vi "svc_FFT with Window.vi"(0 "time signal in [EU]":waveform(dbl), 2 "window":T1=1 items=["None"=0, "Hanning"=1, "Hamming"=2, "Blackman-Harris"=3, "Exact Blackman"=4, "Blackman"=5, "Flat Top"=6, "4 Term B-Harris "=7, "7 Term B-Harris"=8, "Low Sidelobe"=9, "Force"=64, "Exponential"=65, "Blackman Nuttall"=11, "Triangle"=30, "Bartlett-Hanning"=31, "Bohman"=32, "Parzen"=33, "Welch"=34, "Kaiser"=60, "Dolph-Chebyshev"=61, "Gaussian"=62], 5 "error in (no error)":errorcluster) -> (14 "complex spectrum":T8={"complex spectrum response"={"f0"=0.0, "df"=1.0, "complex spectrum"=[]}, "spectrum info"={"channel name"="", "description"="", "x-axis units"=0, "spectral info"={"spectrum type"=enum."Power [Magnitude^2]", "linear/dB"=enum."linear", "window"=0, "window size"=0, "FFT size"=0}, "engineering units"=0, "custom label"="", "dB reference [EU]"=0.0, "peak units"=enum."rms", "weighting filter"=0, "spectral density?"=FALSE, "unit label"="", "spectrum skewed?"=FALSE, "complimentary spectrum units"=enum."none"}} {"spectrum info"."x-axis units" items=["Time (s)"=0, "Frequency-CB (Hz)"=1, "Frequency-CPB (Hz)"=1248, "Frequency-Arbitrary (Hz)"=2357, "Quefrency (s)"=2, "Revolutions (rev)"=3, "Order"=4, "Speed (RPM)"=11, "Speed (rad/s)"=21, "Index"=65535]; "spectrum info"."weighting filter" items=["Linear", "A-weighting", "B-weighting", "C-weighting", "ITU-R 468-4", "Dolby", "CCITT", "C-message", "Wb", "Wc", "Wd", "We", "Wf", "Wh", "Wj", "Wk", "Wm", "AES17 20 kHz lowpass", "AES17 40 kHz lowpass", "AES17 20 kHz highpass", "AES17 40 kHz highpass"]; "spectrum info"."dB reference [EU]" format="%.2f"; "spectrum info"."engineering units" items=["custom..."=0, "V"=1, "A"=21, "C"=30, "pC"=31, "s"=32, "-"=29, "Pa"=2, "N"=20, "g"=3, "m/s^2"=4, "m/s"=5, "m"=6, "mm/s"=12, "mm"=13, "micron/s"=14, "micron"=15, "in/s^2"=7, "in/s"=8, "in"=9, "mil/s"=10, "mil"=11, "rad/s^2"=16, "rad/s"=17, "rad"=18, "deg/s^2"=26, "deg/s"=27, "deg"=28, "RPM"=22, "cycle/s^2"=23, "Hz"=24, "cycle"=25, "strain"=19]; "spectrum info"."spectral info"."window" items=["None "=0, "Hanning"=1, "Hamming"=2, "Blackman-Harris"=3, "Exact Blackman"=4, "Blackman"=5, "Flat Top"=6, "4 Term B-Harris "=7, "7 Term B-Harris"=8, "Low Sidelobe"=9, "Force - Exponential"=10, "Gaussian"=62]; "complex spectrum response"."complex spectrum" format="%.2f"; "complex spectrum response"."df" format="%.2f"; "complex spectrum response"."f0" format="%.2f"}, 19 "error out":errorcluster)   [LabVIEW 2017]
uses:
  <vilib>/addons/_NISVFA/_Shared subVIs/Controls/svc_Spectrum Info.ctl
  <vilib>/addons/_NISVFA/_Shared subVIs/Controls/svc_X-Axis Units.ctl
  <vilib>/addons/_NISVFA/_Shared subVIs/Controls/svc_Spectrum Type.ctl
  <vilib>/addons/_NISVFA/_Shared subVIs/Controls/svc_Engineering Units Text Ring.ctl
  <vilib>/addons/_NISVFA/_Shared subVIs/Controls/svc_Weighting Filter Text Ring.ctl
  <vilib>/addons/_NISVFA/_Shared subVIs/Controls/svc_Complimentary Spectrum Units.ctl
  <vilib>/addons/_NISVFA/_Shared subVIs/Controls/svc_Window.ctl
  <vilib>/Analysis/2dsp.llb/Real FFT.vi
  <vilib>/addons/_NISVFA/_Shared subVIs/Common/svc_Get SV Channel Info.vi
  <vilib>/addons/_NISVFA/_Shared subVIs/Common/svc_Spectrum Units.vi
  <vilib>/Analysis/4window.llb/Force Window.vi
  <vilib>/Analysis/4window.llb/Force Window (DBL).vi
  <vilib>/Analysis/4window.llb/Exponential Window.vi
  <vilib>/Analysis/4window.llb/Exponential Window (DBL).vi
  <vilib>/Utility/error.llb/Error Cluster From Error Code.vi
  <vilib>/Analysis/0measdsp.llb/Scaled Time Domain Window.vi
  <vilib>/Analysis/0measdsp.llb/Scaled Time Domain Window (DBL).vi
  <vilib>/addons/_NISVFA/_Spectrum Processing/subVIs/svfa_Spectrum Info Window to windowTd Type Def.vi
  <vilib>/addons/_NISVFA/_Shared subVIs/Common/svc_Get Weighting Enum and Labels.vi
  <vilib>/addons/_NISVFA/_Shared subVIs/Common/svc_Unit Label Lexical Class.vi
  <vilib>/addons/_NISVFA/_Shared subVIs/Common/svc_Engineering Units to Unit Label.vi
  <vilib>/addons/_NISVFA/_Shared subVIs/Common/svc_Format Value (DBL).vi
  <vilib>/addons/_NISVFA/_Shared subVIs/Common/svc_Channel Info to Spectrum Info.vi
  <vilib>/addons/_NISVFA/_Shared subVIs/Common/svc_Unit Label to Engineering Units.vi
  <vilib>/Analysis/NI_AALPro.lvlib
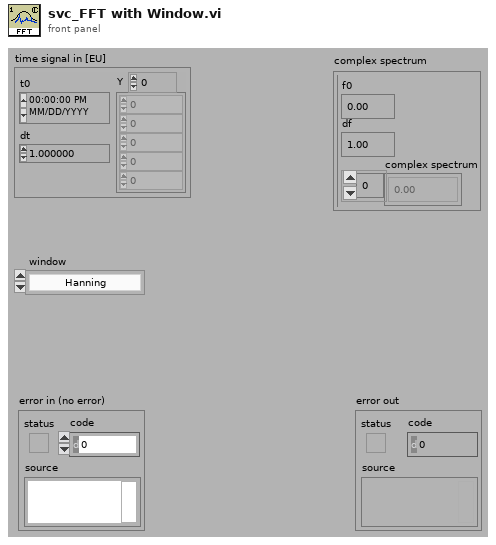
[diagram p1: front panel]
types:
  T1 = typedef "svc_Window.ctl" = u32
  T2 = typedef "svc_Spectrum Info.ctl" = cluster{"channel name":string, "description":string, "x-axis units":T3, "spectral info":cluster{"spectrum type":T4, "linear/dB":enum16{"linear", "dB"}, "window":u16, "window size":i32, "FFT size":i32}, "engineering units":T5, "custom label":string, "dB reference [EU]":dbl, "peak units":enum16{"rms", "peak", "peak-peak"}, "weighting filter":T6, "spectral density?":bool, "unit label":string, "spectrum skewed?":bool, "complimentary spectrum units":T7}
  T3 = typedef "svc_X-Axis Units.ctl" = u16
  T4 = typedef "svc_Spectrum Type.ctl" = enum16{"FFT Spectrum [complex]", "Amplitude [Magnitude]", "Power [Magnitude^2]", "Cross Spectrum [complex]", "Frequency Response [Complex]"}
  T5 = typedef "svc_Engineering Units Text Ring.ctl" = u16
  T6 = typedef "svc_Weighting Filter Text Ring.ctl" = u16
  T7 = typedef "svc_Complimentary Spectrum Units.ctl" = enum16{"none", "radians", "degrees", "cycles", "imaginary"}
  T8 = cluster{"complex spectrum response":cluster{"f0":dbl, "df":dbl, "complex spectrum":cdb[]}, "spectrum info":T2}
  T9 = typedef "NI_AALPro.lvlib/windowTd.ctl" = u32
  T10 = cluster{"complex spectrum":cluster{"f0":dbl, "df":dbl, "complex spectrum":cdb[]}, "spectrum info":T2}
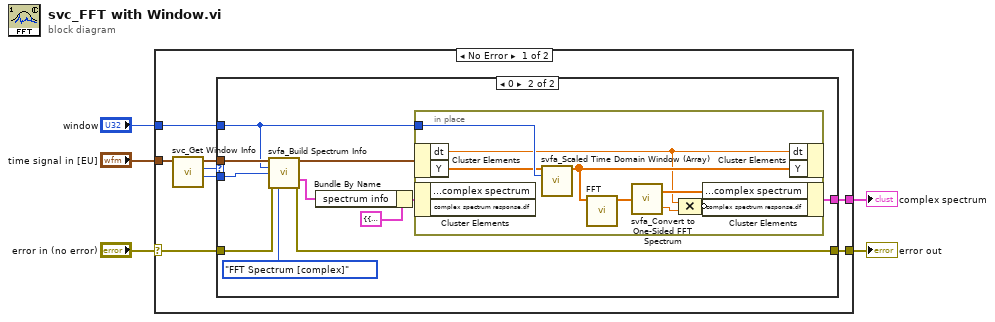
[diagram p0: block diagram]
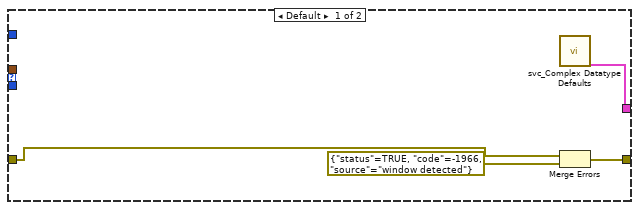
[diagram p2: hidden frame]
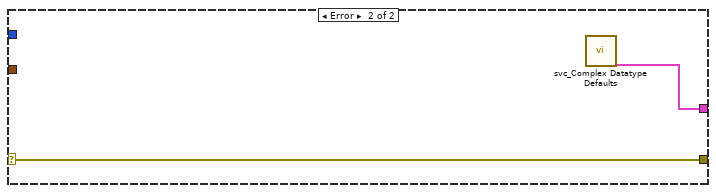
[diagram p3: hidden frame]
diagram:
  n1 = case shown="No Error" "error in (no error)" {
    selector: "error in (no error)" -> [w13 w38]
    tunnel: "time signal in [EU]" -> [w9 _]
    tunnel: [w12 w38] -> w4
    tunnel: [w11 w37] -> w3
    tunnel: "window" -> [w10 _]
    frame No Error {
      n2 = call <vilib>:"svc_Get Window Info.vi"("scaled signal [EU]"=w9) -> ("window size"=w6:i32, "window"=w7:T9, "dup scaled signal [EU]"=w8:waveform(dbl))  [unwired: 6 in, 2 out]
      n3 = case shown="0" w7 {
        tunnel: w13 -> [w16 w28]
        tunnel: [w15 w27] -> w12
        tunnel: [w17 w23] -> w11
        tunnel: w10 -> [_ w20]
        tunnel: w8 -> [_ w26]
        tunnel: w6 -> [_ w19]
        frame Default {
          n4 = call <vilib>:"svc_Complex Datatype Defaults.vi"() -> ("complex spectrum"=w17:T10)  [unwired: 11 in, 8 out]
          n5 = Merge Errors(w16, errorcluster {"status"=TRUE, "code"=-1966, "source"="window detected"} ("error in 2 (no error)")) -> (w15:errorcluster)
        }
        frame 0 {
          n6 = call <vilib>:"svfa_Build Spectrum Info.vi"("scaled signal [EU]"=w26, "window"=w20, "window size"=w19, "error in (no error)"=w28, "spectrum type"=svc_Spectrum_Type."FFT Spectrum [complex]") -> ("dup scaled signal [EU]"=w18:waveform(dbl), "spectrum info out"=w25:T2, "error out"=w27:errorcluster)  [unwired: 7 in, 1 out]
          n7 = Bundle By Name(cluster=T8 {"complex spectrum response"={"f0"=0.0, "df"=1.0, "complex spectrum"=[]}, "spectrum info"={"channel name"="", "description"="", "x-axis units"=0, "spectral info"={"spectrum type"=enum."Power [Magnitude^2]", "linear/dB"=enum."linear", "window"=0, "window size"=0, "FFT size"=0}, "engineering units"=0, "custom label"="", "dB reference [EU]"=0.0, "peak units"=enum."rms", "weighting filter"=0, "spectral density?"=FALSE, "unit label"="", "spectrum skewed?"=FALSE, "complimentary spectrum units"=enum."none"}} ("complex spectrum"), "spectrum info"=w25) -> (w24:T8)
          n8 = in-place {
            in-place-border: w20 -> [w33]
            n9 = in-place-cluster #1(w18) -> ("dt"=w29:dbl, "Y"=w31:dbl[])
            n10 = in-place-cluster #2(w24) -> ()  [unwired: 2 out]
            n11 = call <vilib>:"svfa_Scaled Time Domain Window (Array).vi"("input signal"=w31, "window"=w33) -> ("windowed signal"=w30:dbl[])  [unwired: 8 in, 5 out]
            n12 = call-poly <vilib>:"FFT.vi"("X"=w30) -> ("FFT {X}"=w35:cdb[])  [unwired: 9 in, 1 out]
            n13 = call <vilib>:"svfa_Convert to One-Sided FFT Spectrum.vi"("two-sided FFT spectrum"=w35) -> ("one-sided FFT spectrum"=w34:cdb[], "block size"=w36:dbl)
            n14 = Compound Arithmetic op=MULTIPLY(w29, w36) -> (invert w32:dbl)
            n15 = in-place-cluster #2("complex spectrum response.complex spectrum"=w34, "complex spectrum response.df"=w32) -> (w23:T8)
            n16 = in-place-cluster #1("dt"=w29, "Y"=w30) -> ()  [unwired: 1 out]
          }
        }
      }
    }
    frame Error {
      n17 = call <vilib>:"svc_Complex Datatype Defaults.vi"() -> ("complex spectrum"=w37:T10)  [unwired: 11 in, 8 out]
    }
  }
  "complex spectrum" <- w3
  "error out" <- w4
